vi "SSC DCPower Set Voltage.vi"(0 "DCPower SSC in":T1[](array[typedef]), 5 "Voltage Level, V":dbl, 9 "Voltage Level Range (V)":dbl format="%#_6p", 11 "error in":errorcluster) -> (4 "DCPower SSC out":T1[](array[typedef]), 15 "error out":errorcluster)   [LabVIEW 2019]
doc: "This Vi configure voltage with previous current limit setting"
uses:
  Instrument Control/DCPower/SSC DCPower/SSC DCPower.ctl
  <instrlib>/niDCPower/nidcpower.llb/niDCPower Output Function.ctl
  <instrlib>/niDCPower/nidcpower.llb/niDCPower Source Mode.ctl
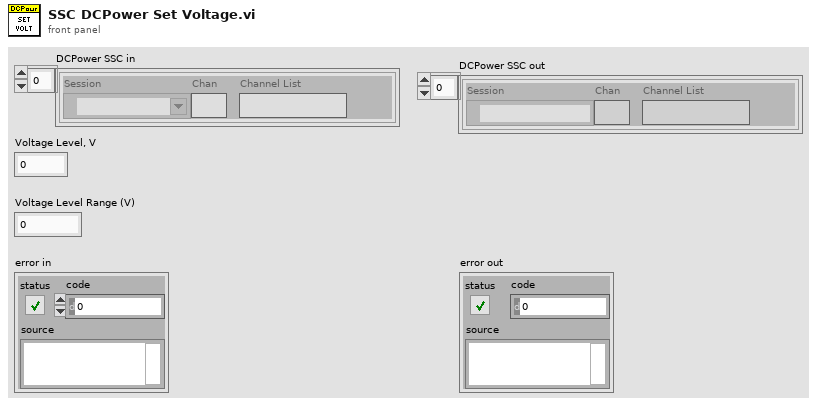
[diagram p1: front panel]
types:
  T1 = typedef "SSC DCPower.ctl" = cluster{"Session":refnum<k15>, "Chan":string, "Channel List":string}
  T2 = typedef "niDCPower Source Mode.ctl" = i32
  T3 = typedef "niDCPower Output Function.ctl" = i32
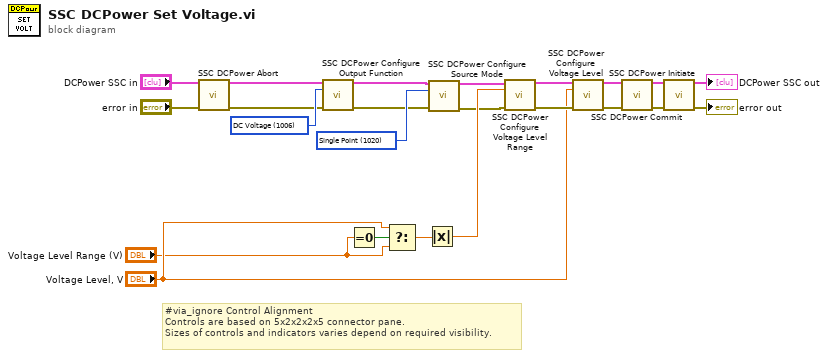
[diagram p0: block diagram]
diagram:
  w5 = T2 1020 items=["Single Point"=1020, "Sequence"=1021] ("Source Mode")
  w23 = T3 1006 items=["DC Voltage"=1006, "DC Current"=1007, "Pulse Voltage"=1049, "Pulse Current"=1050] ("Output Function")
  # "#via_ignore Control Alignment\nControls are based on 5x2x2x2x5 connector pane.\nSizes of controls and indicators varies depend on required visibility."
  n1 = call "SSC DCPower Abort.vi"("DCPower SSC in"="DCPower SSC in", "error in"="error in") -> ("DCPower SSC out"=w16:T1[], "error out"=w18:errorcluster)  [unwired: 12 in]
  n2 = call "SSC DCPower Configure Output Function.vi"("DCPower SSC in"=w16, "Output Function"=w23, "error in"=w18) -> ("DCPower SSC out"=w4:T1[], "error out"=w3:errorcluster)  [unwired: 11 in]
  n3 = Equal To 0?(x="Voltage Level Range (V)") -> (x = 0?=w10:bool)
  n4 = Select(t="Voltage Level, V", s=w10, f="Voltage Level Range (V)") -> (s? t:f=w7:dbl)
  n5 = Absolute Value(x=w7) -> (abs(x)=w6:dbl)
  n6 = call "SSC DCPower Configure Source Mode.vi"("DCPower SSC in"=w4, "Source Mode"=w5, "error in"=w3) -> ("DCPower SSC out"=w2:T1[], "error out"=w1:errorcluster)  [unwired: 11 in]
  n7 = call "SSC DCPower Configure Voltage Level Range.vi"("DCPower SSC in"=w2, "Voltage Level Range (V)"=w6, "error in"=w1) -> ("DCPower SSC out"=w21:T1[], "error out"=w20:errorcluster)  [unwired: 11 in]
  n8 = call "SSC DCPower Configure Voltage Level.vi"("DCPower SSC in"=w21, "Voltage Level (V)"="Voltage Level, V", "error in"=w20) -> ("DCPower SSC out"=w14:T1[], "error out"=w19:errorcluster)  [unwired: 11 in]
  n9 = call "SSC DCPower Commit.vi"("DCPower SSC in"=w14, "error in"=w19) -> ("DCPower SSC out"=w12:T1[], "error out"=w15:errorcluster)  [unwired: 12 in]
  n10 = call "SSC DCPower Initiate.vi"("DCPower SSC in"=w12, "error in"=w15) -> ("DCPower SSC out"=→"DCPower SSC out":T1[], "error out"=→"error out":errorcluster)  [unwired: 12 in]
